vi "SMO.BasicByRef.TestLauncher.vi"() -> ()   [LabVIEW 2019, in "SMO.BasicByRef.lvclass"]
doc: "JKI State Machine Objects (SMO) 1.0.0.5\nJKI - JKI\nCopyright (c) 2016, JKI"
uses:
  SMO.BasicByRef.lvclass
  vi.lib/JKI/JKI SMO/SMO/Typedefs/SMOState --Enum.ctl
  C:/Users/Patrick/Documents/GitHub/Test (LV2019)/lv-venv/lv.lib/vi.lib/JKI/JKI SMO/SMO/SMO.lvclass
  Typedefs/Value.ctl
  vi.lib/JKI/JKI SMO/SMO/SMO.lvclass
panel:
  out "State":T1
  out "New Value Event":string
  in  "Send":bool
  in  "Value":string
  out "error out":errorcluster
  in  "Stop":bool
  # "Basic SMO byRef Test Launcher"
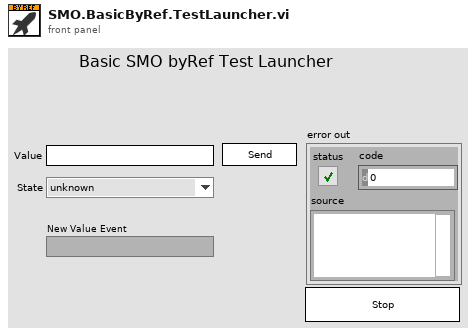
[diagram p1: front panel]
types:
  T1 = typedef "SMO.lvclass/SMOState --Enum.ctl" = enum16{"unknown", "Created", "Started", "Stopped"}
  T2 = typedef "SMO.BasicByRef.lvclass/Value.ctl" = string
  T3 = typedef "SMO.BasicByRef.lvclass/PublicEvents--Cluster.ctl" = cluster{"Value Changed":refnum<user-event>}
  T4 = typedef "SMO.lvclass/Public Events.ctl" = cluster{"Error":refnum<user-event>, "State":refnum<user-event>, "Reserve State":refnum<user-event>}
  T5 = cluster{"Event Registration Refnum":refnum<event-registration>}
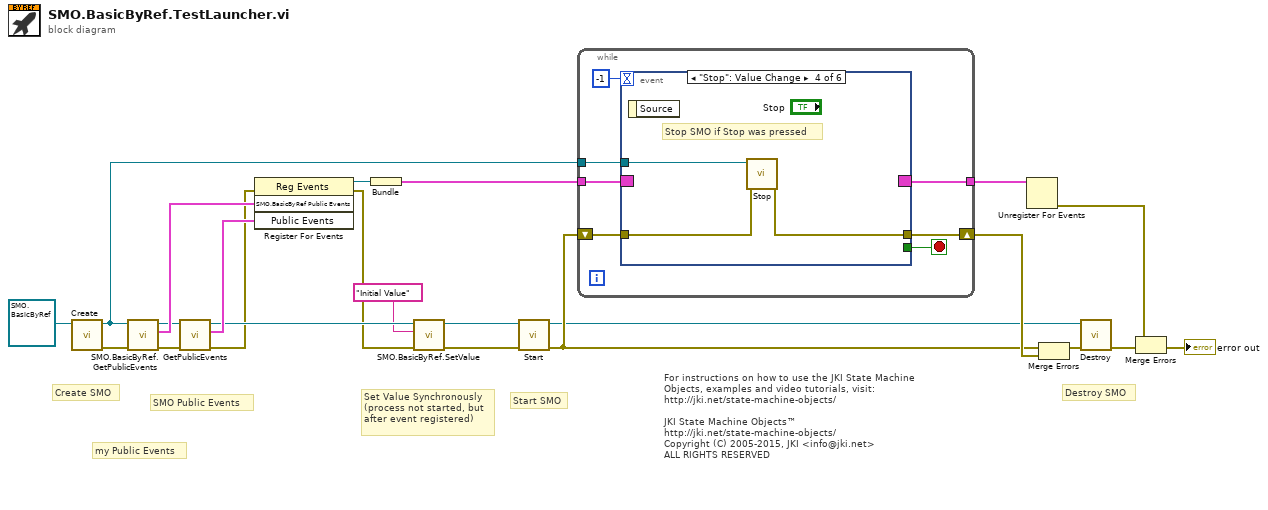
[diagram p0: block diagram]
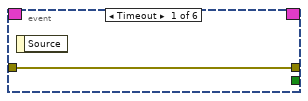
[diagram p2: hidden frame]
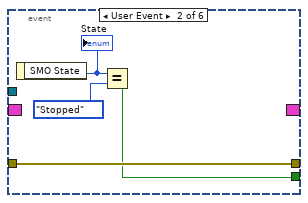
[diagram p3: hidden frame]
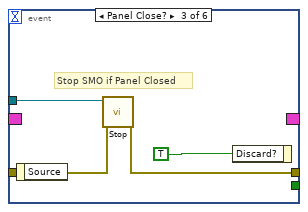
[diagram p4: hidden frame]
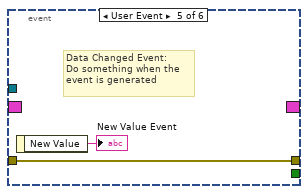
[diagram p5: hidden frame]
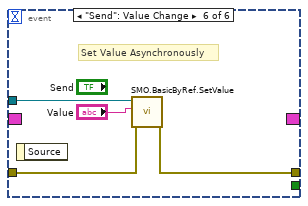
[diagram p6: hidden frame]
diagram:
  # "Set Value Synchronously\n(process not started, but\nafter event registered)"
  # "SMO Public Events"
  # "For instructions on how to use the JKI State Machine Objects, examples and video tutorials, visit:\nhttp://jki.net/state-machine-objects/\n\nJKI State Machine Objects™\nhttp://jki.net/state-machine-objects/\nCopyright (C) 2005-2015, JKI <info@jki.net>\nALL RIGHTS RESERVED"
  # "my Public Events"
  # "Start SMO"
  # "Destroy SMO"
  # "Create SMO"
  n1 = call "Create.vi"("SMO"=refnum<class "SMO.BasicByRef.lvclass"> refnum ("SMO.Template.lvclass")) -> ("error out"=w15:errorcluster, "SMO out"=w12:refnum<class "SMO.BasicByRef.lvclass">)  [unwired: 8 in, 1 out]
  n2 = call "SMO.BasicByRef.GetPublicEvents.vi"("error in (no error)"=w15, "SMO.BasicByRef"=w12) -> ("error out"=w10:errorcluster, "SMO.BasicByRef Public Events"=w14:T3, "SMO.BasicByRef out"=w11:refnum<class "SMO.BasicByRef.lvclass">)  [unwired: 7 in]
  n3 = call "GetPublicEvents.vi"("error in (no error)"=w10, "SMO"=w11) -> ("error out"=w4:errorcluster, "Public Events"=w9:T4, "SMO out"=w8:refnum<class "SMO.BasicByRef.lvclass">)  [unwired: 7 in]
  n4 = register-events(error in=w4, w14, w9) -> (reference out=w13:refnum<event-registration>, error out=w3:errorcluster)  [unwired: 1 in]
  n5 = Bundle("Event Registration Refnum"=w13) -> (w22:T5)  [unwired: 1 in]
  n6 = call "SMO.BasicByRef.SetValue.vi"("error in (no error)"=w3, "Value"=T2 "Initial Value", "SMO.BasicByRef"=w8) -> ("error out"=w6:errorcluster, "SMO.BasicByRef out"=w7:refnum<class "SMO.BasicByRef.lvclass">)  [unwired: 6 in, 1 out]
  n7 = call "Start.vi"("error in (no error)"=w6, "SMO"=w7) -> ("error out"=w16:errorcluster, "SMO out"=w1:refnum<class "SMO.BasicByRef.lvclass">)  [unwired: 8 in]
  n8 = while {
    shift-right: [w29] -> w21
    shift-left: w16 -> [w28]
    tunnel: w22 -> [w27]
    tunnel: [w26] -> w23
    tunnel: w12 -> [w25]
    stop <- w30 stop-if-true
    n9 = event shown="[3] \"Stop\": Value Change" {
      selector: w27 -> [_ _ _ _ _ _]
      dyn-events: [_ _ _ _ _ _] -> w26
      timeout: -1 -> [_ _ _ _ _ _]
      tunnel: [_ w32 _ _ _ _] -> w30
      tunnel: w25 -> [_ _ w39 w42 _ w48]
      tunnel: [w31 w35 w38 w41 w44 w45] -> w29
      tunnel: w28 -> [w31 w35 w37 w40 w44 w46]
      event Timeout {
        n10 = event-data() -> ()  [unwired: 1 in, 1 out]
      }
      event User Event {
        n11 = event-data() -> ("SMO State"=w34:T1)  [unwired: 1 in]
        "State" <- w34
        n12 = Equal?(x=w34, y=SMOState_--Enum."Stopped") -> (x = y?=w32:bool)
      }
      event Panel Close? {
        # "Stop SMO if Panel Closed"
        n13 = event-data() -> ()  [unwired: 1 in, 1 out]
        n14 = call "Stop.vi"("error in (no error)"=w37, "SMO"=w39) -> ("error out"=w38:errorcluster)  [unwired: 8 in, 1 out]
        n15 = event-data("Discard?"=TRUE ("OK")) -> ()  [unwired: 1 in, 1 out]
      }
      event "Stop": Value Change {
        # "Stop SMO if Stop was pressed"
        n16 = event-data() -> ()  [unwired: 1 in, 1 out]
        n17 = call "Stop.vi"("error in (no error)"=w40, "SMO"=w42) -> ("error out"=w41:errorcluster)  [unwired: 8 in, 1 out]
      }
      event User Event {
        # "Data Changed Event:\nDo something when the\nevent is generated"
        n18 = event-data() -> ("New Value"=→"New Value Event":string)  [unwired: 1 in]
      }
      event "Send": Value Change {
        # "Set Value Asynchronously"
        n19 = event-data() -> ()  [unwired: 1 in, 1 out]
        n20 = call "SMO.BasicByRef.SetValue.vi"("error in (no error)"=w46, "Value"="Value", "SMO.BasicByRef"=w48) -> ("error out"=w45:errorcluster)  [unwired: 6 in, 2 out]
      }
    }
  }
  n21 = Unregister For Events(event registration refnum=w23) -> (error out=w20:errorcluster)  [unwired: 1 in]
  n22 = Merge Errors(w16, w21) -> (w2:errorcluster)
  n23 = call "Destroy.vi"("error in (no error)"=w2, "SMO"=w1) -> ("error out"=w18:errorcluster)  [unwired: 9 in]
  n24 = Merge Errors(w20, w18) -> (→"error out":errorcluster)
